vi "write IP configuration.vi"(0 "identifier":string, 5 "IP":string, 7 "subnet_mask":string, 9 "gateway":string, 11 "error in (no error)":errorcluster) -> (3 "function return":u32, 4 "identifier out":string, 6 "IP out":string, 8 "subnet_mask out":string, 10 "gateway out":string, 15 "error out":errorcluster)   [LabVIEW 2015, in "XGL_DPP.lvlib"]
doc: "EXTERN DECLSPEC unsigned int CALL_CONV write_IP_configuration(char* identifier, char* IP, char* subnet_mask, char* gateway);"
uses:
  XGL_DPP.lvlib
  D:/Scanning Software_Demokritos_2015_v6/libs/XGL_DPP.dll
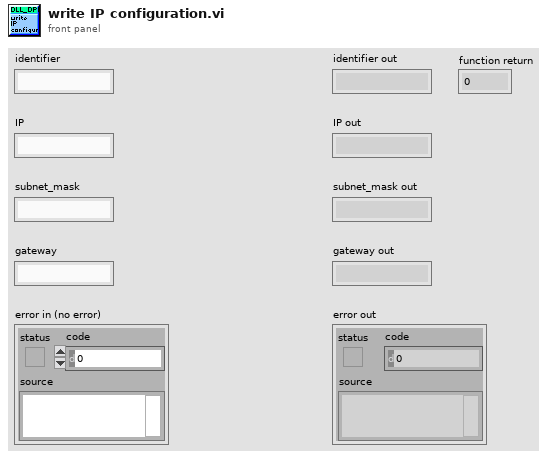
[diagram p1: front panel]
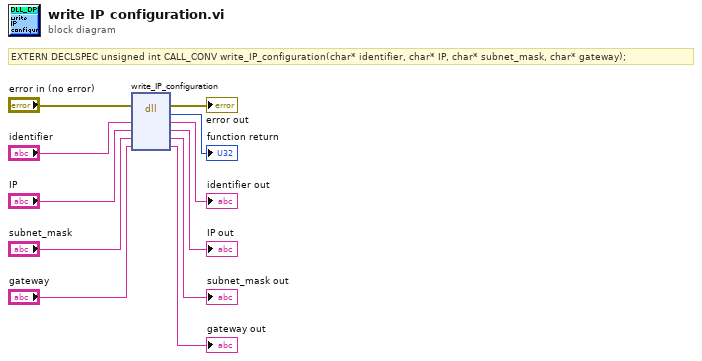
[diagram p0: block diagram]
diagram:
  # "EXTERN DECLSPEC unsigned int CALL_CONV write_IP_configuration(char* identifier, char* IP, char* subnet_mask, char* gateway);"
  n1 = dll-call lib="D:/Scanning Software_Demokritos_2015_v6/libs/XGL_DPP.*" fn="write_IP_configuration"(error in="error in (no error)", "identifier"="identifier", "IP"="IP", "subnet_mask"="subnet_mask", "gateway"="gateway") -> (error out=→"error out":errorcluster, "return type"=→"function return":u32, "identifier"=→"identifier out":string, "IP"=→"IP out":string, "subnet_mask"=→"subnet_mask out":string, "gateway"=→"gateway out":string)  [unwired: 2 in, 1 out]
